vi "end Sw--sq C1.vi"(8 "Command Info In":T2, 10 "end Sw--sq C1":T1={"1a"=-90.0, "1d"=-48.0, "1s"=-0.5, "2d"=67.25, "2s"=0.75}, 11 "Switch":string) -> (0 "Command Info Out":T2)   [LabVIEW 2017]
uses:
  <vilib>/Rock Robotics/WPI/Framework/Command Status Info.ctl
  <vilib>/Rock Robotics/WPI/Framework/Completion Status.ctl
  <vilib>/Rock Robotics/WPI/Framework/Completion Notifier.ctl
  Block Clusters/end Sw--sq C1.ctl
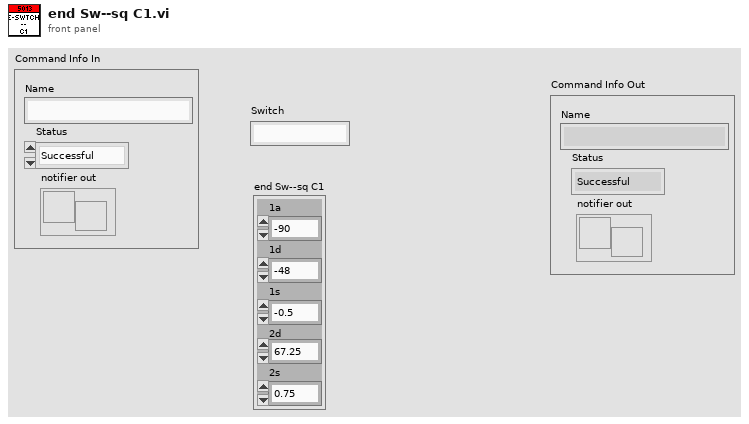
[diagram p1: front panel]
types:
  T1 = typedef "end Sw--sq C1.ctl" = cluster{"1a":dbl, "1d":dbl, "1s":dbl, "2d":dbl, "2s":dbl}
  T2 = typedef "Command Status Info.ctl" = cluster{"Name":string, "Status":T3, "notifier out":T4}
  T3 = typedef "Completion Status.ctl" = enum16{"Successful", "Aborted", "Incomplete"}
  T4 = typedef "Completion Notifier.ctl" = refnum<notifier>
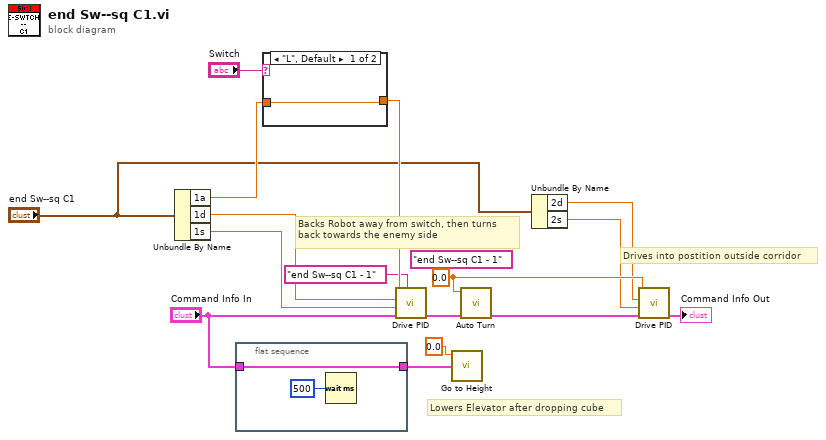
[diagram p0: block diagram]
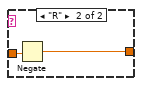
[diagram p2: hidden frame]
diagram:
  (unwired) "end Sw--sq C1 - 1" ("Description")
  w6 = 0.0 ("Target Angle")
  # "Drives into postition outside corridor"
  # "Backs Robot away from switch, then turns back towards the enemy side"
  # "Lowers Elevator after dropping cube"
  n1 = Unbundle By Name("end Sw--sq C1") -> ("1a"=w9:dbl, "1d"=w8:dbl, "1s"=w7:dbl)
  n2 = flat-sequence {
    tunnel: "Command Info In" -> [w17]
    tunnel: [w17] -> w11
    frame #0 {
      n3 = Wait (ms)(milliseconds to wait=u32 500 ("millisecond timer value")) -> ()  [unwired: 1 out]
    }
  }
  n4 = case shown="\"L\", Default" "Switch" {
    tunnel: [w19 w21] -> w10
    tunnel: w9 -> [w19 w20]
    frame "L", Default {
    }
    frame "R" {
      n5 = Negate(x=w20) -> (-x=w21:dbl)
    }
  }
  n6 = call "Drive PID.vi"("Description"="end Sw--sq C1 - 1", "Command Info In"="Command Info In", "Speed"=w7, "Distance"=w8, "Target Angle"=w10) -> ("Command Info Out"=w15:T2)  [unwired: 6 in]
  n7 = call "Go to Height.vi"("Command Info In"=w11, "Target Height (in)"=0.0) -> ()  [unwired: 9 in, 1 out]
  n8 = call "Auto Turn.vi"("Command Info In"=w15, "Target Angle"=w6) -> ("Command Info Out"=w14:T2)  [unwired: 9 in]
  n9 = Unbundle By Name("end Sw--sq C1") -> ("2d"=w4:dbl, "2s"=w3:dbl)
  n10 = call "Drive PID.vi"("Command Info In"=w14, "Speed"=w3, "Distance"=w4, "Target Angle"=w6) -> ("Command Info Out"=→"Command Info Out":T2)  [unwired: 7 in]
